vi "外观.vi"(0 "Data In":T5 caption="数据输入", 2 "Display State In":T3={"显示位数"=6, "小数位数"=0} caption="显示状态输入", 3 "Container State":T4 caption="容器状态") -> (6 "Data Out":T5 caption="数据输出", 7 "Display State Out":T3={"显示位数"=6, "小数位数"=0} caption="显示状态输出", 8 "Action":T2 caption="动作")   [LabVIEW 2013, in "数码管.xctl"]
uses:
  <vilib>/_xctls/Container State.ctl
  <vilib>/_xctls/Action.ctl
  <vilib>/_xctls/XControlSupport.lvlib
panel:
  out "arr":T1[](array[typedef])
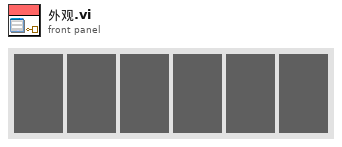
[diagram p1: front panel]
types:
  T1 = typedef "数码管.xctl/LED_small_white.ctl" = u16
  T2 = typedef "XControlSupport.lvlib/Action.ctl" = cluster{"Data Changed?":bool, "State Changed?":bool, "Action Name":string}
  T3 = typedef "数码管.xctl/数码管.ctl" = cluster{"显示位数":u8, "小数位数":u8}
  T4 = typedef "XControlSupport.lvlib/Container State.ctl" = cluster{"Indicator?":bool, "Run Mode?":bool, " Refnum":refnum<vi>}
  T5 = typedef "数码管.xctl/数据.ctl" = dbl
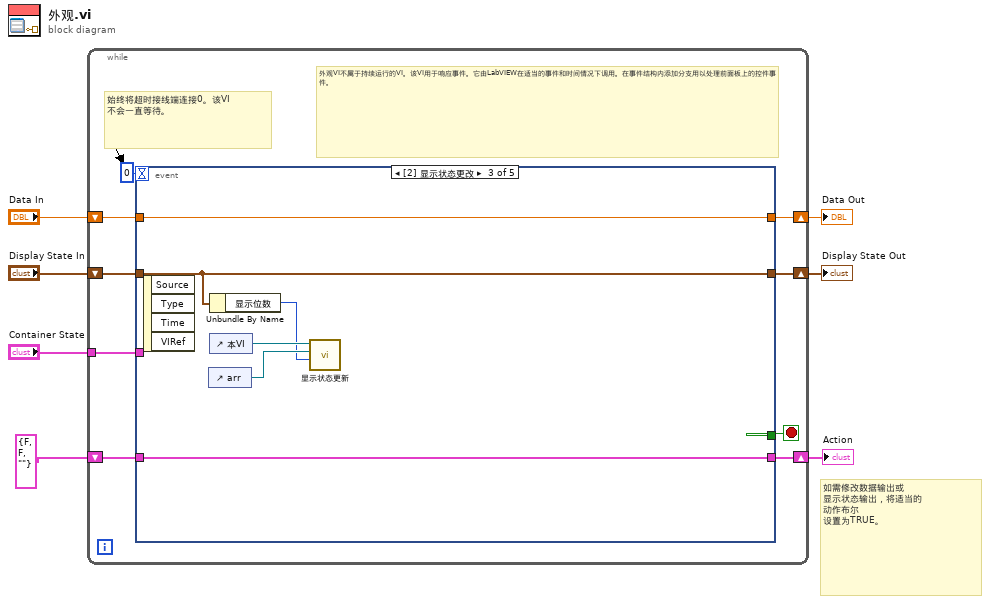
[diagram p0: block diagram]
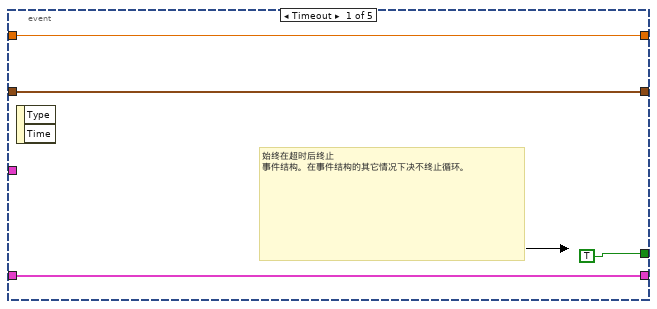
[diagram p2: hidden frame]
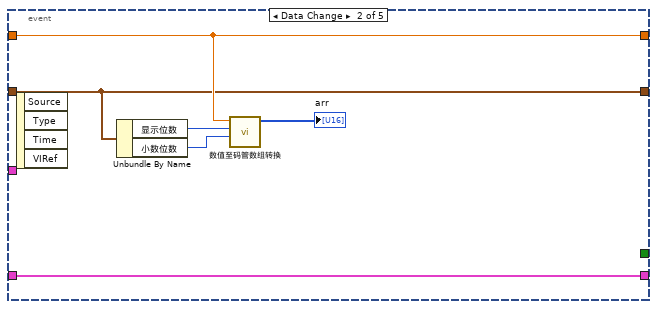
[diagram p3: hidden frame]
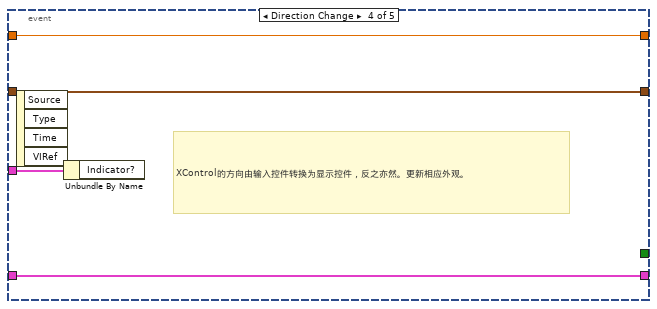
[diagram p4: hidden frame]
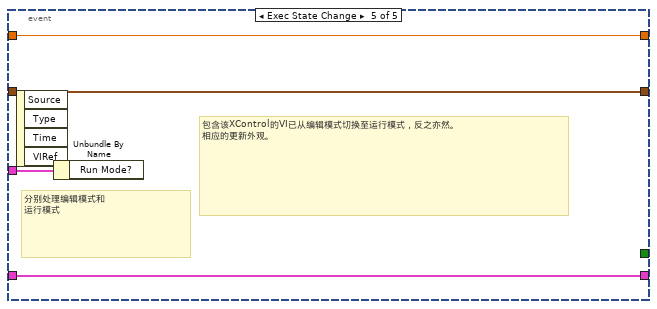
[diagram p5: hidden frame]
diagram:
  # "如需修改数据输出或\n显示状态输出，将适当的\n动作布尔\n设置为TRUE。"
  n1 = while {
    shift-right: [w15] -> w4
    shift-left: "Display State In" -> [w16]
    tunnel: "Container State" -> [w12]
    shift-right: [w10] -> w7
    shift-left: "Data In" -> [w11]
    shift-right: [w8] -> w2
    shift-left: T2 {"Data Changed?"=FALSE, "State Changed?"=FALSE, "Action Name"=""} ("Action") -> [w9]
    stop <- w14 stop-if-true
    # "外观VI不属于持续运行的VI。该VI用于响应事件。它由LabVIEW在适当的事件和时间情况下调用。在事件结构内添加分支用以处理前面板上的控件事件。"
    # "始终将超时接线端连接0。该VI\n不会一直等待。"
    n2 = event shown="[2] 显示状态更改" {
      selector: _ -> [_ _ _ _ _]
      dyn-events: _ -> [_ _ _ _ _]
      timeout: 0 -> [_ _ _ _ _]
      tunnel: w16 -> [w18 w23 w30 w35 w39]
      tunnel: [w18 w23 w30 w35 w39] -> w15
      tunnel: [TRUE _ _ _ _] -> w14
      tunnel: w12 -> [_ _ _ w36 w40]
      tunnel: w11 -> [w17 w25 w32 w34 w38]
      tunnel: [w17 w25 w32 w34 w38] -> w10
      tunnel: [w19 w26 w31 w33 w37] -> w8
      tunnel: w9 -> [w19 w26 w31 w33 w37]
      event Timeout {
        # "始终在超时后终止\n事件结构。在事件结构的其它情况下决不终止循环。"
        n3 = event-data() -> ()  [unwired: 1 in, 2 out]
      }
      event Data Change {
        n4 = event-data() -> ()  [unwired: 1 in, 4 out]
        n5 = Unbundle By Name(w23) -> ("显示位数"=w21:u8, "小数位数"=w22:u8)
        n6 = call "数值至码管数组转换.vi"("小数位数"=w22, "显示位数"=w21, "数值"=w25) -> ("数组"=→"arr":u16[])  [unwired: 8 in]
      }
      event Display State Change {
        n7 = event-data() -> ()  [unwired: 1 in, 4 out]
        n8 = control-ref of="arr"() -> (w28:refnum<vi>)
        n9 = Unbundle By Name(w30) -> ("显示位数"=w27:u8)
        n10 = control-ref of="本VI"() -> (w29:refnum<vi>)
        n11 = call "显示状态更新.vi"("显示位数"=w27, "码管数组引用"=w28, "外观vi引用"=w29) -> ()  [unwired: 9 in]
      }
      event Direction Change {
        # "XControl的方向由输入控件转换为显示控件，反之亦然。更新相应外观。"
        n12 = event-data() -> ()  [unwired: 1 in, 4 out]
        n13 = Unbundle By Name(w36) -> ()  [unwired: 1 out]
      }
      event Exec State Change {
        # "包含该XControl的VI已从编辑模式切换至运行模式，反之亦然。\n相应的更新外观。"
        # "分别处理编辑模式和\n运行模式"
        n14 = event-data() -> ()  [unwired: 1 in, 4 out]
        n15 = Unbundle By Name(w40) -> ()  [unwired: 1 out]
      }
    }
  }
  "Display State Out" <- w4
  "Data Out" <- w7
  "Action" <- w2
